vi "Vi Tester Time Measurement Runner.vi"() -> ()   [LabVIEW 2018]
panel:
  in  "All Test":bool
  out "VI Tester In Progress":bool
  out "VI Tester report":string
  out "VI Tester Testing time (seconds)":dbl
  in  "Action Update Heater State":bool=TRUE
  in  "Action Update Set Point":bool=TRUE
  in  "Action Update Ramp Rate":bool=TRUE
  in  "Multiplier of runs":i32=10
  out "No. of Tests":i32=10
  # "VI Tester"
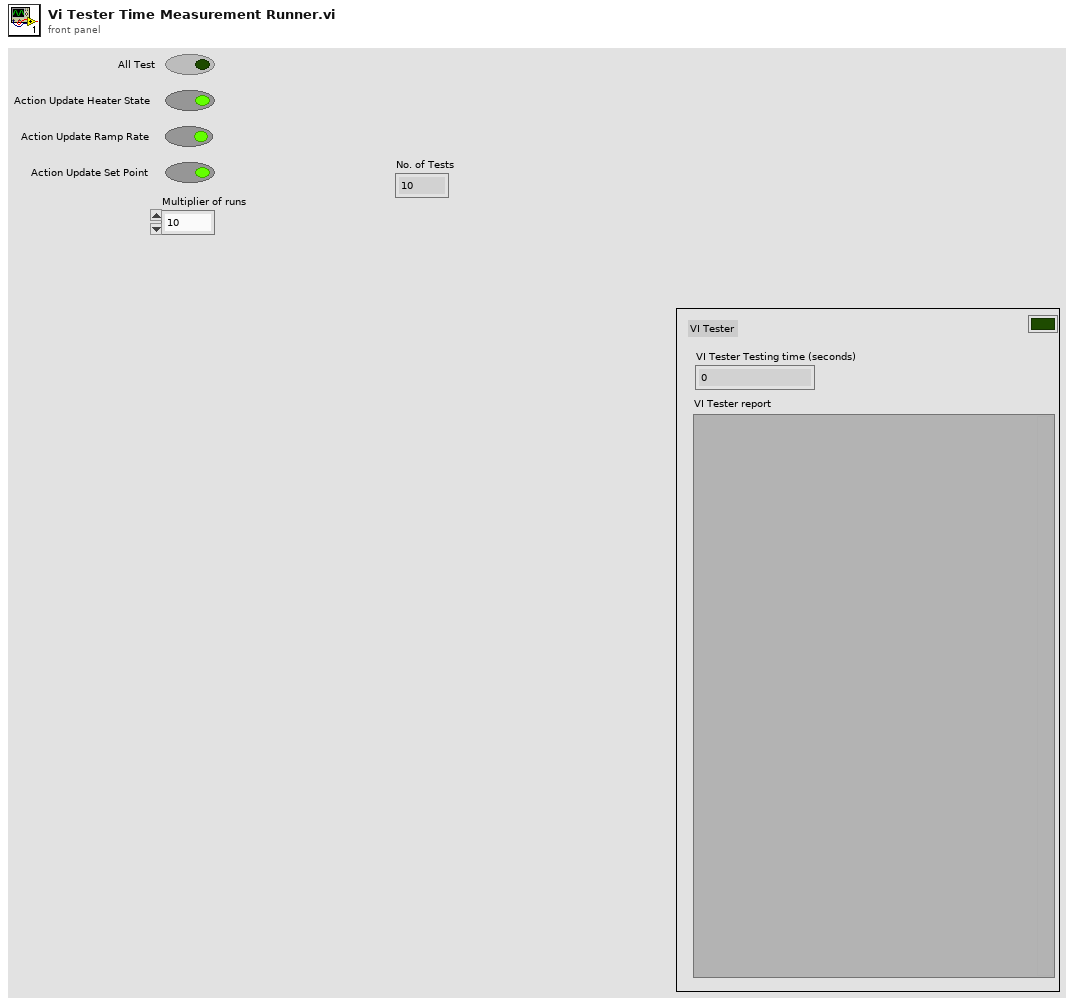
[diagram p1: front panel]
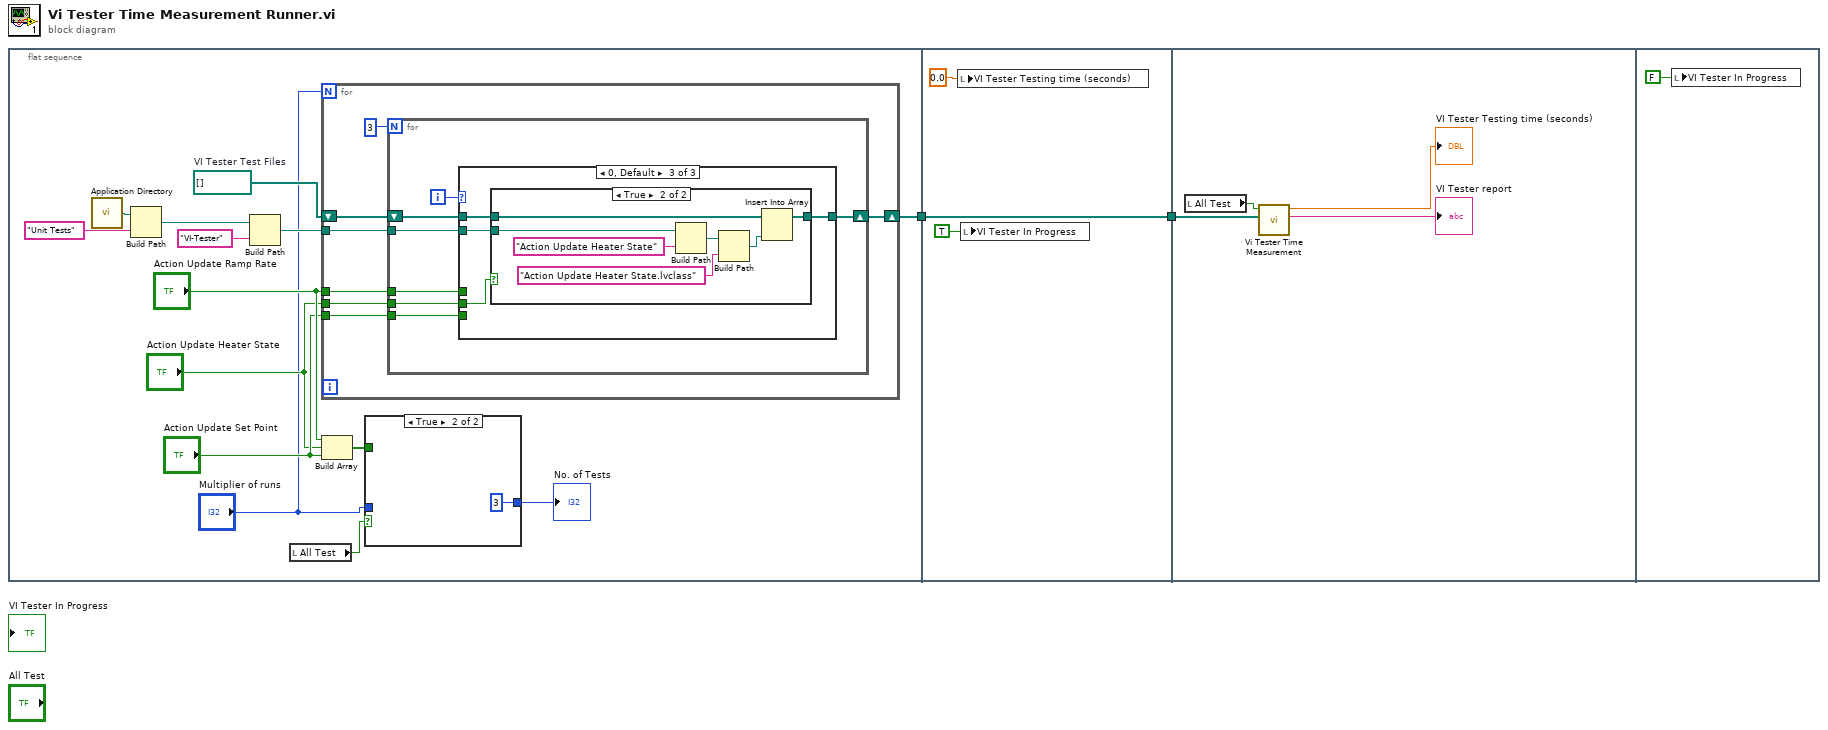
[diagram p0: block diagram]
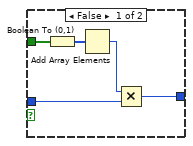
[diagram p2: hidden frame]
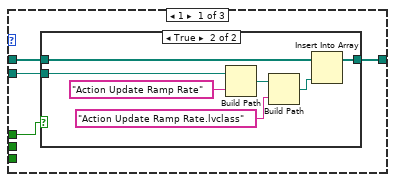
[diagram p3: hidden frame]
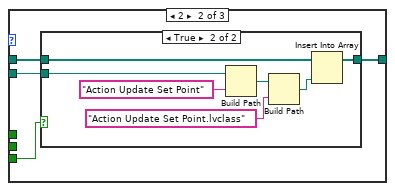
[diagram p5: hidden frame]
diagram:
  n1 = flat-sequence {
    tunnel: [w11] -> w2
    tunnel: [w74] -> w1
    tunnel: w2 -> [w74]
    tunnel: w1 -> [w76]
    frame #0 {
      w16 = path[] []  # VI Tester Test Files
      n2 = call <vilib>:"Application Directory.vi"() -> ("Application Directory"=w15:path)
      n3 = Build Path(base path=w15, name or relative path="Unit Tests") -> (appended path=w12:path)
      n4 = Build Path(base path=w12, name or relative path="VI-Tester") -> (appended path=w10:path)
      n5 = local read "All Test"() -> (w9:bool)
      n6 = for {
        N: "Multiplier of runs" -> [_]
        tunnel: "Action Update Heater State" -> [w29]
        tunnel: "Action Update Ramp Rate" -> [w27]
        tunnel: "Action Update Set Point" -> [w26]
        tunnel: w10 -> [w24]
        shift-right: [w25] -> w11
        shift-left: w16 -> [w28]
        n7 = for {
          N: 3 -> [_]
          tunnel: w29 -> [w36]
          tunnel: w24 -> [w33]
          shift-right: [w34] -> w25
          shift-left: w28 -> [w35]
          tunnel: w27 -> [w31]
          tunnel: w26 -> [w30]
          i -> [w32]
          n8 = case shown="0, Default" w32 {
            tunnel: w36 -> [_ _ w64]
            tunnel: w35 -> [w40 w51 w63]
            tunnel: [w38 w49 w62] -> w34
            tunnel: w33 -> [w39 w50 w61]
            tunnel: w31 -> [w37 _ _]
            tunnel: w30 -> [_ w52 _]
            frame 1 {
              n9 = case shown="True" w37 {
                tunnel: w40 -> [w41 w48]
                tunnel: [w41 w47] -> w38
                tunnel: w39 -> [_ w45]
                frame False {
                }
                frame True {
                  n10 = Build Path(base path=w45, name or relative path="Action Update Ramp Rate") -> (appended path=w43:path)
                  n11 = Build Path(base path=w43, name or relative path="Action Update Ramp Rate.lvclass") -> (appended path=w42:path)
                  n12 = Insert Into Array(array=w48, new element=w42) -> (w47:path[])  [unwired: 1 in]
                }
              }
            }
            frame 2 {
              n13 = case shown="True" w52 {
                tunnel: [w53 w60] -> w49
                tunnel: w50 -> [_ w58]
                tunnel: w51 -> [w53 w57]
                frame False {
                }
                frame True {
                  n14 = Build Path(base path=w58, name or relative path="Action Update Set Point") -> (appended path=w55:path)
                  n15 = Build Path(base path=w55, name or relative path="Action Update Set Point.lvclass") -> (appended path=w54:path)
                  n16 = Insert Into Array(array=w57, new element=w54) -> (w60:path[])  [unwired: 1 in]
                }
              }
            }
            frame 0, Default {
              n17 = case shown="True" w64 {
                tunnel: w63 -> [w65 w72]
                tunnel: [w65 w71] -> w62
                tunnel: w61 -> [_ w69]
                frame False {
                }
                frame True {
                  n18 = Build Path(base path=w69, name or relative path="Action Update Heater State") -> (appended path=w67:path)
                  n19 = Build Path(base path=w67, name or relative path="Action Update Heater State.lvclass") -> (appended path=w68:path)
                  n20 = Insert Into Array(array=w72, new element=w68) -> (w71:path[])  [unwired: 1 in]
                }
              }
            }
          }
        }
      }
      n21 = Build Array("Action Update Ramp Rate", "Action Update Heater State", "Action Update Set Point") -> (w8:bool[])
      n22 = case shown="True" w9 {
        tunnel: w8 -> [w21 _]
        tunnel: "Multiplier of runs" -> [w19 _]
        tunnel: [w17 3 ("Multiplier of runs")] -> w3
        frame False {
          n23 = Boolean To (0,1)(Boolean=w21) -> (0, 1=w20:i16[])
          n24 = Add Array Elements(numeric array=w20) -> (sum=w18:i16)
          n25 = Multiply(x=w18, y=w19) -> (x*y=w17:i32)
        }
        frame True {
        }
      }
      "No. of Tests" <- w3
    }
    frame #1 {
      n26 = local write "VI Tester Testing time (seconds)"(0.0 ("VI Tester Testing time (seconds)")) -> ()
      n27 = local write "VI Tester In Progress"(TRUE) -> ()
    }
    frame #2 {
      n28 = local read "All Test"() -> (w77:bool)
      n29 = call "Vi Tester Time Measurement.vi"("test file paths"=w76, "All Test"=w77) -> ("VI Tester report"=→"VI Tester report":string, "VI Tester Testing time (seconds)"=→"VI Tester Testing time (seconds)":dbl)  [unwired: 8 in]
    }
    frame #3 {
      n30 = local write "VI Tester In Progress"(FALSE ("ICov In Progress")) -> ()
    }
  }
